vi "MoAgSy_Host_GPG_getPubKey_p.vi"(0 "MoAgSy_Host":refnum<class "MoAgSy_Host.lvclass">, 5 "error in (no error)":errorcluster) -> (14 "dup MoAgSy_Host":refnum<class "MoAgSy_Host.lvclass">, 16 "public Key":string, 19 "error out":errorcluster)   [LabVIEW 2009, in "MoAgSy.lvlib" / "MoAgSy_Host.lvclass"]
doc: "<b>private</b> read hosts public key\n\nF.Berck@gsi.de\nGSI Darmstadt 2009"
uses:
  MoAgSy_Host.lvclass
  MoAgSy_Host.lvclass/MoAgSy_Host.ctl
  MoAgSy_GPG/MoAgSy_GPG.lvclass
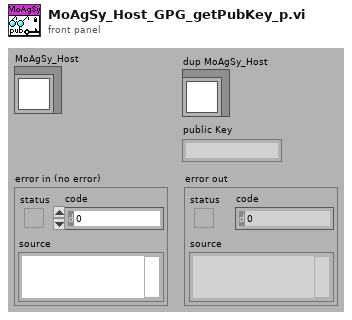
[diagram p1: front panel]
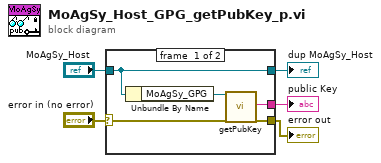
[diagram p0: block diagram]
diagram:
  n1 = case shown="No Error" "error in (no error)" {
    selector: "error in (no error)" -> [w10 w12]
    tunnel: [w9 w12] -> w4
    tunnel: "MoAgSy_Host" -> [w8 w11]
    tunnel: [w8 w11] -> w2
    tunnel: [w6 _] -> w1
    frame #0 {
      n2 = Unbundle By Name(w8) -> ("MoAgSy_GPG"=w7:refnum<class "MoAgSy_GPG.lvclass">)
      n3 = call-dynamic "getPubKey.vi"("HGF_GPG.lvclass in"=w7, "error in (no error)"=w10) -> ("public Key"=w6:string, "error out"=w9:errorcluster)  [unwired: 15 in, 1 out]
    }
    frame #1 {
    }
  }
  "error out" <- w4
  "dup MoAgSy_Host" <- w2
  "public Key" <- w1
